vi "Transform Point.vi"(1 "Point to Transform":cluster{"X":dbl, "Y":dbl}, 2 "Transformation Matrix":T1) -> (0 "Transformed Point":cluster{"X":dbl, "Y":dbl})   [LabVIEW 2020]
doc: "Transforms a point based on a transformation matrix."
uses:
  <vilib>/Analysis/Matrix/Datatypes/RealMatrix.ctl
  <vilib>/Analysis/baseanly.llb/Real A x B.vi
  <vilib>/Analysis/Matrix/Numeric/Conversions/Array To Matrix - RA.vi
  <vilib>/Analysis/Matrix/NI_Matrix.lvlib
  <vilib>/Analysis/NI_AALBase.lvlib
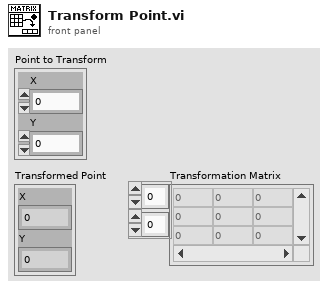
[diagram p1: front panel]
types:
  T1 = typedef "NI_Matrix.lvlib/RealMatrix.ctl" = dbl[][]
  T2 = cluster{"Real Matrix Element":dbl, "Real Matrix Element":dbl}
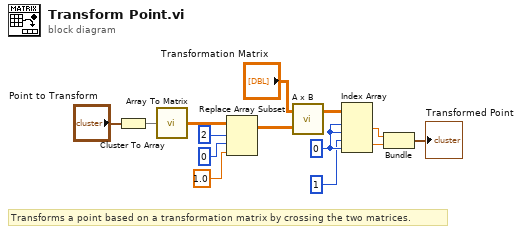
[diagram p0: block diagram]
diagram:
  w5 = 0 ("index (row)")
  # "Transforms a point based on a transformation matrix by crossing the two matrices."
  n1 = Cluster To Array(cluster="Point to Transform") -> (array=w13:dbl[])
  n2 = call-poly <vilib>:"Array To Matrix.vi"("Real 1D Array"=w13) -> ("Real Matrix (Column Vector)"=w12:T1)
  n3 = Replace Array Subset(array=w12, new element=1.0 ("new element/submatrix"), index (row)=2 ("disabled index (row)"), index (col)=0 ("disabled index (col)")) -> (w8:T1)
  n4 = call-poly <vilib>:"A x B.vi"("B"=w8, "A"="Transformation Matrix") -> ("A x B"=w6:T1)  [unwired: 1 out]
  n5 = Index Array(array=w6, index (row) #1=w5, index (col) #1=w5, index (row) #2=1 ("index (row)"), index (col) #2=w5) -> (element #1=w3:dbl, element #2=w2:dbl)
  n6 = Bundle("Real Matrix Element"=w3, "Real Matrix Element"=w2) -> (→"Transformed Point":T2)  [unwired: 1 in]
